vi "StatsToPlugin.vi"(10 "Stats":T1(array[cluster]) {"Min" format="%0.2f"; "Max" format="%0.2f"; "mean(5Maxs)" format="%0.2f"; "mean(5Mins)" format="%0.2f"; "SD(Cp)" format="%0.2f"; "meanCp" format="%0.2f"}, 11 "AdditionalNote":string) -> (1 "Plug in values":string[](array[string]), 2 "Plug in titles":string[](array[string]))   [LabVIEW 2011]
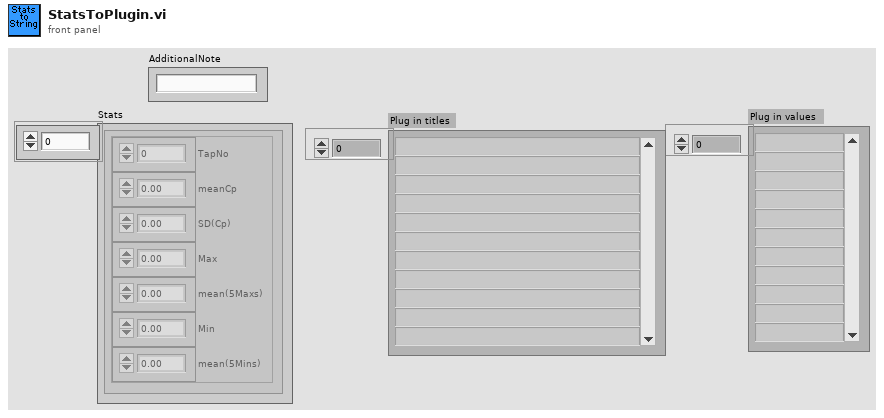
[diagram p1: front panel]
types:
  T1 = cluster{"TapNo":i32, "meanCp":dbl, "SD(Cp)":dbl, "Max":dbl, "mean(5Maxs)":dbl, "Min":dbl, "mean(5Mins)":dbl}[]
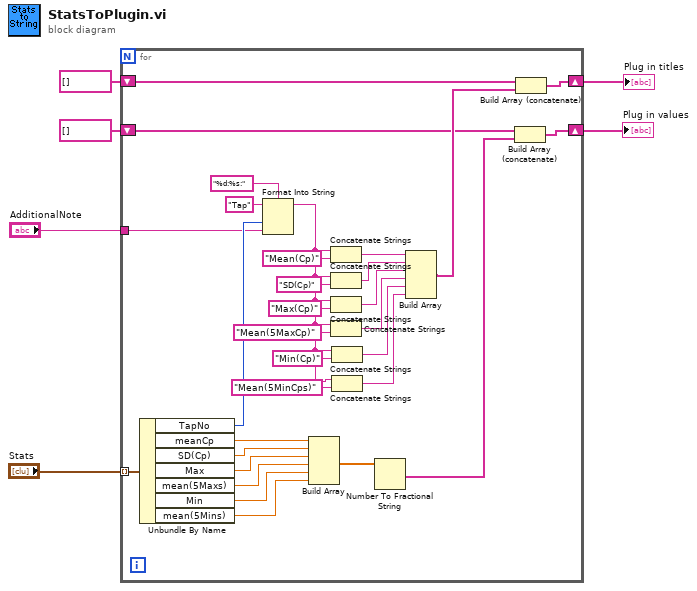
[diagram p0: block diagram]
diagram:
  n1 = for {
    tunnel: "Stats" -> [w37] mode=indexing
    tunnel: "AdditionalNote" -> [w27]
    shift-right: [w12] -> w4
    shift-left: string[] [] -> [w10]
    shift-right: [w9] -> w3
    shift-left: string[] [] -> [w8]
    n2 = Unbundle By Name(w37) -> ("TapNo"=w30:i32, "meanCp"=w36:dbl, "SD(Cp)"=w35:dbl, "Max"=w34:dbl, "mean(5Maxs)"=w33:dbl, "Min"=w32:dbl, "mean(5Mins)"=w31:dbl)
    n3 = Format Into String(format string="%d:%s:", initial string="Tap", w30, w27) -> (resulting string=w26:string)  [unwired: 1 in, 1 out]
    n4 = Build Array(w36, w35, w34, w33, w32, w31) -> (w19:dbl[])
    n5 = Concatenate Strings(w26, "Mean(Cp)" ("string")) -> (w25:string)
    n6 = Concatenate Strings(w26, "SD(Cp)" ("string")) -> (w24:string)
    n7 = Concatenate Strings(w26, "Max(Cp)" ("string")) -> (w23:string)
    n8 = Concatenate Strings(w26, "Mean(5MaxCp)" ("string")) -> (w22:string)
    n9 = Concatenate Strings(w26, "Min(Cp)" ("string")) -> (w21:string)
    n10 = Concatenate Strings(w26, "Mean(5MinCps)" ("string")) -> (w20:string)
    n11 = Number To Fractional String(number=w19) -> (F-format string=w7:string[])  [unwired: 3 in]
    n12 = Build Array(w25, w24, w23, w22, w21, w20) -> (w11:string[])
    n13 = Build Array (concatenate)(w8, w7) -> (w9:string[])
    n14 = Build Array (concatenate)(w10, w11) -> (w12:string[])
  }
  "Plug in titles" <- w4
  "Plug in values" <- w3
